vi "P3AT_Ini_Pose_Msg.vi"(8 "error in (no error)":errorcluster caption="错误输入（无错误）", 10 "值(信号)":T1, 11 "States.lvlib:Localize.lvclass":refnum<class "Localize.lvclass">) -> (0 "error out":errorcluster caption="错误输出", 3 "Process State out":refnum<class "State Actor.lvclass">)   [LabVIEW 2014, in "States.lvlib" / "Localize.lvclass"]
uses:
  Localize.lvclass
  <vilib>/NI/Actors/State Actor/State Actor/State Actor.lvclass
  <vilib>/ActorFramework/Message Enqueuer/Message Enqueuer.lvclass/Message Enqueuer.ctl
  <vilib>/ActorFramework/Message Enqueuer/Enqueue.vi
  <vilib>/ActorFramework/Message Priority Queue/Priority Enqueue.vi
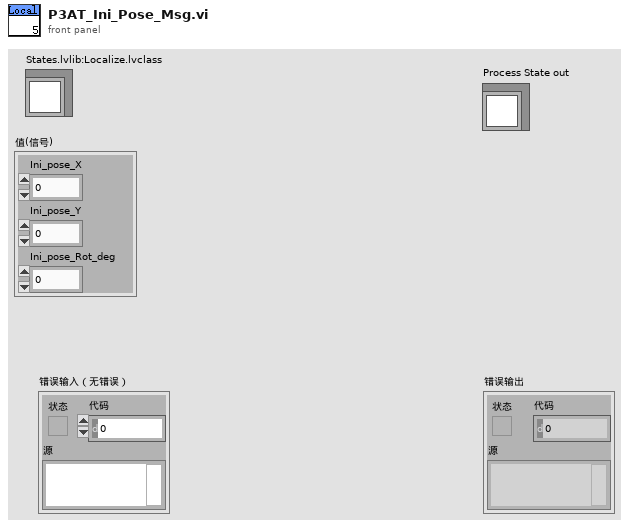
[diagram p1: front panel]
types:
  T1 = cluster{"Ini_pose_X":dbl, "Ini_pose_Y":dbl, "Ini_pose_Rot_deg":dbl}
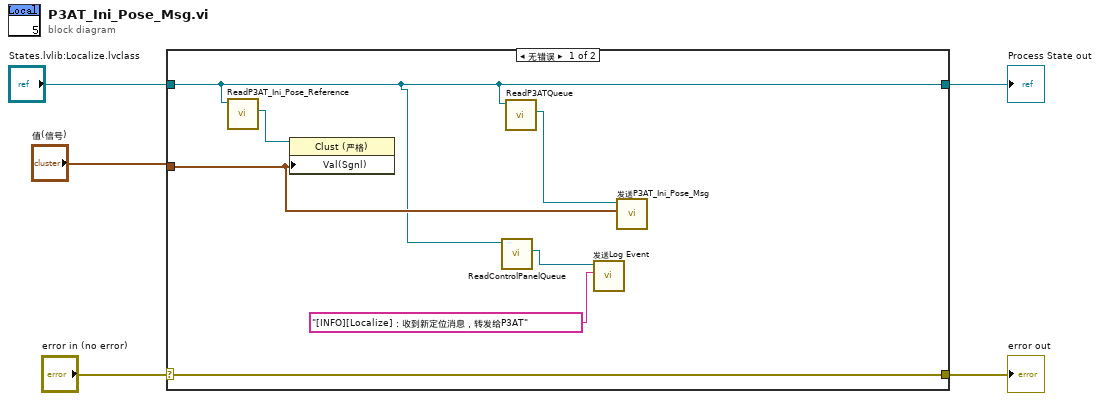
[diagram p0: block diagram]
diagram:
  n1 = case shown="无错误" "error in (no error)" {
    selector: "error in (no error)" -> [w12 w13]
    tunnel: [w12 w13] -> w4
    tunnel: [w7 w14] -> w3
    tunnel: "States.lvlib:Localize.lvclass" -> [w7 w14]
    tunnel: "值(信号)" -> [w9 _]
    frame No Error {
      n2 = call-dynamic "ReadP3AT_Ini_Pose_Reference.vi"("CoordinatorState输入"=w7) -> ("P3AT_Ini_Pose_Reference"=w10:refnum<vi>)  [unwired: 8 in, 2 out]
      n3 = property class="Clust (严格)"(reference=w10, "Val(Sgnl)"=w9) -> ()  [unwired: 1 in, 2 out]
      n4 = call-dynamic "ReadControlPanelQueue.vi"("CoordinatorState输入"=w7) -> ("操作者框架:消息待入队列"=w6:refnum<class "Message Enqueuer.lvclass">)  [unwired: 8 in, 2 out]
      n5 = call-dynamic "ReadP3ATQueue.vi"("CoordinatorState输入"=w7) -> ("操作者框架:消息待入队列"=w11:refnum<class "Message Enqueuer.lvclass">)  [unwired: 8 in, 2 out]
      n6 = call "发送Log Event.vi"("Event Text"="[INFO][Localize]：收到新定位消息，转发给P3AT", "消息待入队列"=w6) -> ()  [unwired: 8 in, 2 out]
      n7 = call "发送P3AT_Ini_Pose_Msg.vi"("值(信号)"=w9, "消息待入队列"=w11) -> ()  [unwired: 8 in, 2 out]
    }
    frame Error {
    }
  }
  "error out" <- w4
  "Process State out" <- w3
